vi "Query Quanta Transmitter Serial Number.vi"(0 "RS232 Port In":refnum<visa-resource-name>, 1 "Sensor Address In":string, 7 "Error In (No Error)":errorcluster) -> (20 "RS232 Port Out":refnum<visa-resource-name>, 21 "Address Out":string, 22 "SDI-12 Compatibility Number":dbl, 23 "Company Name":string, 24 "Sensor Model Number":string, 25 "Sensor Version":string, 26 "Serial Number/MISC":string, 27 "Error Out":errorcluster)   [LabVIEW 2015, in "SDI-12.lvlib"]
doc: "Sends an SDI-12 Send Identification Command, and returns the various attributes from the sensor's response.\n\nThe total size by the sensor must be 22-35 in size (inclusive), or this VI will return an error."
uses:
  SDI-12.lvlib
panel:
  out "read buffer":string
  in  "write buffer":string="XSN!"
  out "length":i32
  # "(c) 2008 National Instruments.  ALL RIGHTS RESERVED."
  # "The following are required,\nor are optional, for the sensors\nto respond with:"
  # "Length:"
  # "REQUIRED:"
  # "1 FIXED"
  # "REQUIRED:"
  # "2 FIXED"
  # "REQUIRED:"
  # "8 FIXED"
  # "REQUIRED:"
  # "6 FIXED"
  # "REQUIRED:"
  # "3 FIXED"
  # "OPTIONAL:"
  # "1-13 Inclusive Variable"
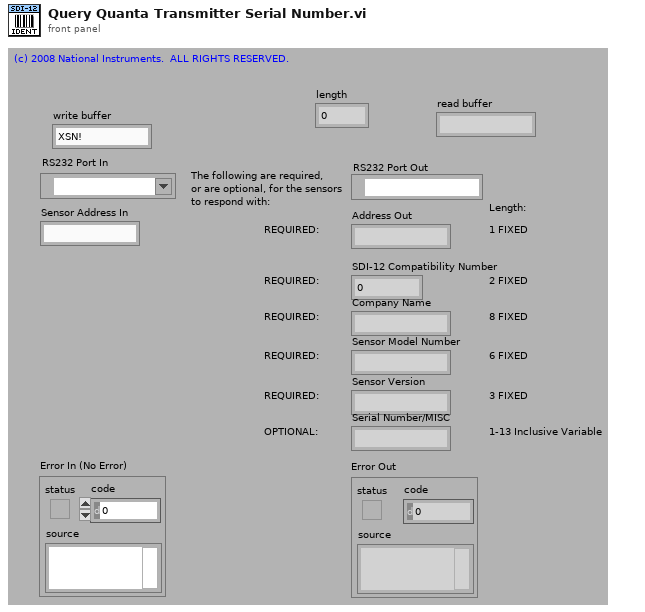
[diagram p1: front panel]
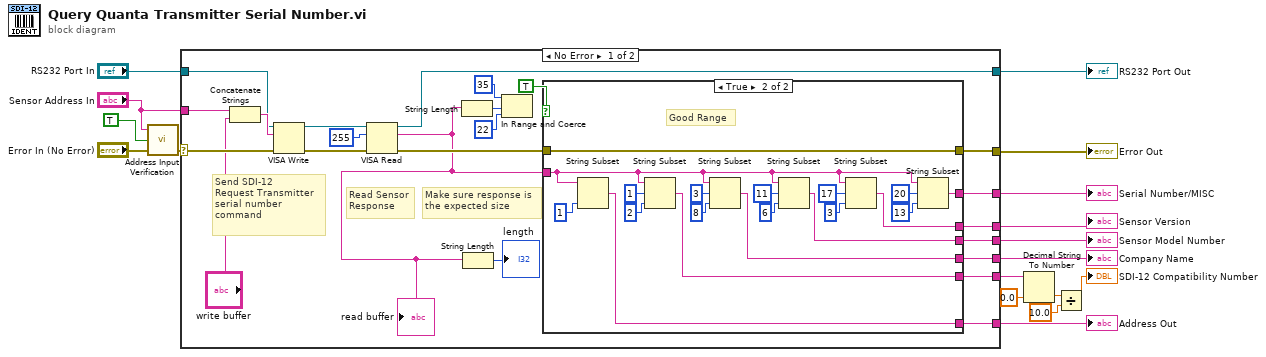
[diagram p0: block diagram]
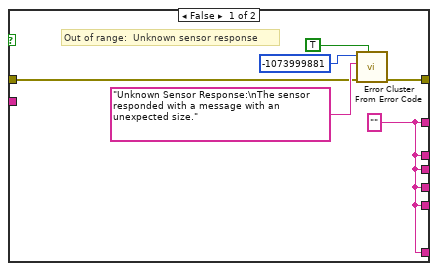
[diagram p2: hidden frame]
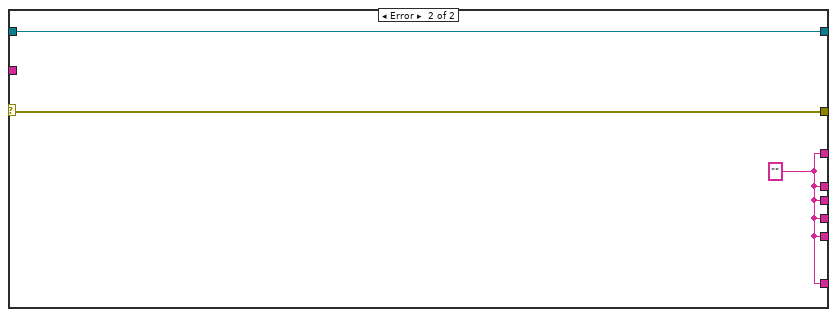
[diagram p3: hidden frame]
diagram:
  n1 = call "Address Input Verification.vi"("Error In (No Error)"="Error In (No Error)", "Error if Bad? (True)"=TRUE ("error if bad? (True)"), "Sensor Address In (a)"="Sensor Address In") -> ("Error Out"=w15:errorcluster)  [unwired: 1 in, 1 out]
  n2 = case shown="No Error" w15 {
    selector: w15 -> [w37 w68]
    tunnel: [w27 w68] -> w17
    tunnel: "Sensor Address In" -> [w36 _]
    tunnel: "RS232 Port In" -> [w33 w67]
    tunnel: [w32 w67] -> w12
    tunnel: [w26 w66] -> w10
    tunnel: [w25 w66] -> w9
    tunnel: [w24 w66] -> w8
    tunnel: [w23 w66] -> w7
    tunnel: [w22 w66] -> w5
    tunnel: [w21 w66] -> w6
    frame No Error {
      # "Make sure response is\nthe expected size"
      # "Send SDI-12 \nRequest Transmitter \nserial number \ncommand"
      # "Read Sensor\nResponse"
      n3 = Concatenate Strings(w36, "write buffer") -> (w34:string)
      n4 = VISA Write(VISA resource name=w33, write buffer=w34, error in (no error)=w37) -> (VISA resource name out=w40:refnum<visa-resource-name>, error out=w39:errorcluster)  [unwired: 1 out]
      n5 = VISA Read(VISA resource name=w40, byte count=u32 255, error in (no error)=w39) -> (VISA resource name out=w32:refnum<visa-resource-name>, read buffer=w20:string, error out=w28:errorcluster)  [unwired: 1 out]
      "read buffer" <- w20
      n6 = String Length(string=w20) -> (length=w29:i32)
      n7 = String Length(string=w20) -> (length=→"length":i32)
      n8 = In Range and Coerce(upper limit=35, x=w29, lower limit=22) -> ()  [unwired: 2 out]
      n9 = case shown="True" TRUE {
        tunnel: w28 -> [w42 w53]
        tunnel: [w43 w53] -> w27
        tunnel: w20 -> [_ w59]
        tunnel: [w41 w52] -> w26
        tunnel: [w41 w51] -> w25
        tunnel: [w41 w50] -> w24
        tunnel: [w41 w49] -> w23
        tunnel: [w41 w48] -> w22
        tunnel: [w41 w47] -> w21
        frame False {
          w41 = "" ("read buffer")
          # "Out of range:  Unknown sensor response"
          n10 = call <vilib>:"Error Cluster From Error Code.vi"("show call chain? (False)"=TRUE, "error in (no error)"=w42, "error message (\"\")"="Unknown Sensor Response:\nThe sensor responded with a message with an unexpected size." ("error message (\"\")"), "error code (0)"=-1073999881) -> ("error out"=w43:errorcluster)  [unwired: 5 in]
        }
        frame True {
          # "Good Range"
          n11 = String Subset(string=w59, length (rest)=1 ("length (rest)")) -> (substring=w47:string)  [unwired: 1 in]
          n12 = String Subset(string=w59, offset (0)=1, length (rest)=2 ("length (rest)")) -> (substring=w48:string)
          n13 = String Subset(string=w59, offset (0)=3, length (rest)=8 ("length (rest)")) -> (substring=w49:string)
          n14 = String Subset(string=w59, offset (0)=11, length (rest)=6 ("length (rest)")) -> (substring=w50:string)
          n15 = String Subset(string=w59, offset (0)=17, length (rest)=3 ("length (rest)")) -> (substring=w51:string)
          n16 = String Subset(string=w59, offset (0)=20, length (rest)=13 ("length (rest)")) -> (substring=w52:string)
        }
      }
    }
    frame Error {
      w66 = "" ("read buffer")
    }
  }
  "Error Out" <- w17
  "RS232 Port Out" <- w12
  "Serial Number/MISC" <- w10
  "Sensor Version" <- w9
  "Sensor Model Number" <- w8
  "Company Name" <- w7
  "Address Out" <- w6
  n17 = Decimal String To Number(string=w5, default (0L)=0.0 ("default (0 I32)")) -> (number=w2:dbl)  [unwired: 1 in, 1 out]
  n18 = Divide(x=w2, y=10.0) -> (x/y=→"SDI-12 Compatibility Number":dbl)
